vi "SaveProjectForPreviousVersion.vi"(8 "error in (no error) 2":errorcluster, 9 "Version":string, 10 "Target Path":path, 11 "Project Path":path) -> (0 "error out":errorcluster)   [LabVIEW 2019]
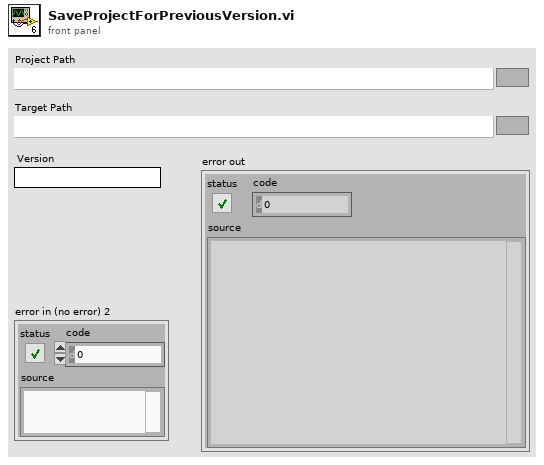
[diagram p1: front panel]
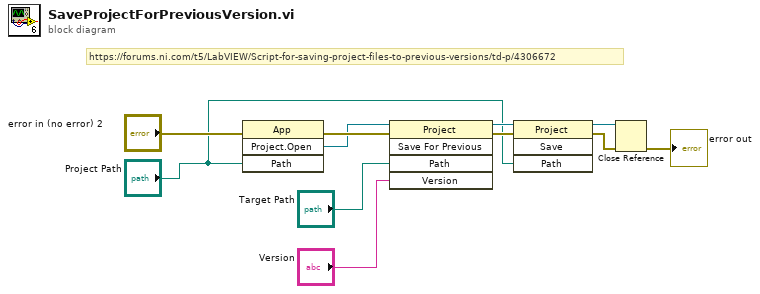
[diagram p0: block diagram]
diagram:
  # "https://forums.ni.com/t5/LabVIEW/Script-for-saving-project-files-to-previous-versions/td-p/4306672"
  n1 = invoke class="App" method="Project.Open"(error in="error in (no error) 2", "Path"="Project Path") -> (error out=w11:errorcluster, "Project:Open"=w10:refnum<vi>)  [unwired: 2 in, 2 out]
  n2 = invoke class="Project" method="Save For Previous"(reference=w10, error in=w11, "Path"="Target Path", "Version"="Version") -> (reference out=w9:refnum<vi>, error out=w3:errorcluster)  [unwired: 1 in, 3 out]
  n3 = invoke class="Project" method="Save"(reference=w9, error in=w3, "Path"="Project Path") -> (reference out=w4:refnum<vi>, error out=w2:errorcluster)  [unwired: 1 in, 2 out]
  n4 = Close Reference(reference=w4, error in (no error)=w2) -> (error out=→"error out":errorcluster)
